vi "SystemNode_Create.vi"(0 "reference":refnum<class "SystemNode.lvclass">, 5 "error in (no error)":errorcluster) -> (14 "reference out":refnum<class "SystemNode.lvclass">, 19 "error out":errorcluster)   [LabVIEW 2016, in "SystemNode.lvclass"]
doc: "Creates and initializes a new SystemNode object.\n\nThis object should be destroyed using a SystemNode destructor VI or a virtual base class destructor VI.\n\n[GOOP 2.1]"
uses:
  <resource>/Framework/Providers/Open_GDS/UML/SystemNode_class/SystemNode.lvclass
  C:/Program Files (x86)/National Instruments/LabVIEW 2016/resource/Framework/Providers/Open_GDS/UML/RectangularNode_class/RectangularNode.lvclass
  <resource>/Framework/Providers/Open_GDS/UML/RectangularNode_class/RectangularNode.lvclass
  <resource>/Framework/Providers/Open_GDS/UML/MultiLineString_class/MultiLineString.lvclass
panel:
  # "The input reference should only\nbe wired when this method is called\nby a sub class constructor."
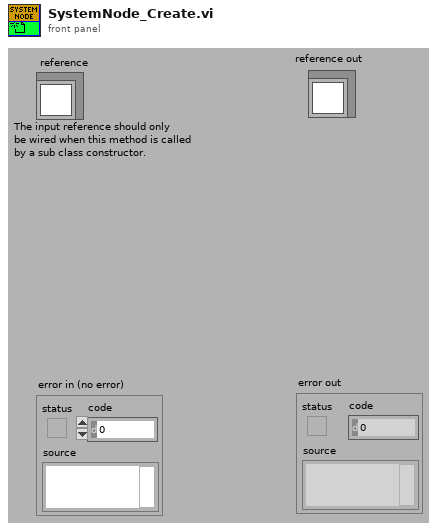
[diagram p1: front panel]
types:
  T1 = typedef "SystemNode.lvclass/ObjectAttributes.ctl" = cluster{"contents":refnum<class "MultiLineString.lvclass">, "DEFAULT_WIDTH":i32, "DEFAULT_HEIGHT":i32, "NAME_GAP":i32, "XGAP":i32, "YGAP":i32}
  T2 = typedef "RectangularNode.lvclass/ObjectAttributes.ctl" = cluster{"bounds":T3}
  T3 = typedef "Rectangle Rectangle2D.ctl" = cluster{"x":dbl, "y":dbl, "width":dbl, "height":dbl}
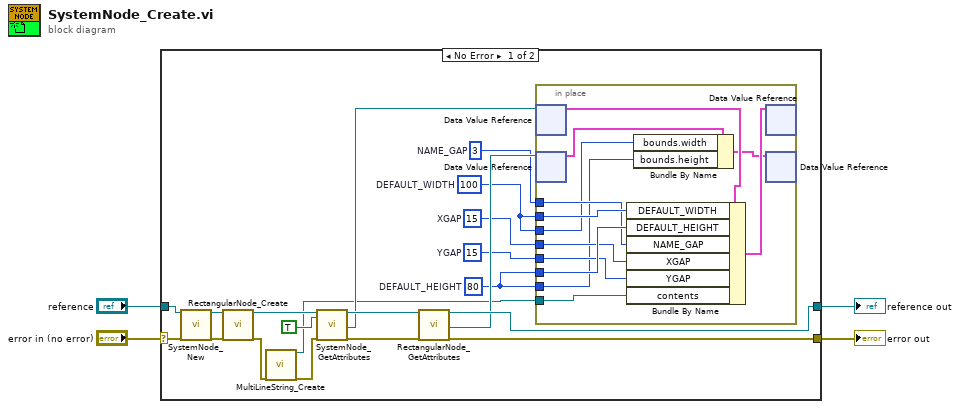
[diagram p0: block diagram]
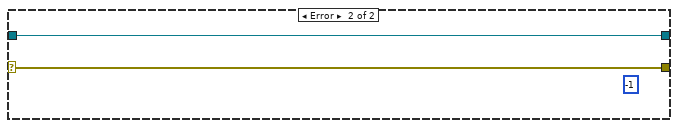
[diagram p2: hidden frame]
diagram:
  n1 = case shown="No Error" "error in (no error)" {
    selector: "error in (no error)" -> [w24 w38]
    tunnel: [w20 w37] -> w4
    tunnel: [w19 w38] -> w3
    tunnel: "reference" -> [w23 w37]
    frame No Error {
      w8 = 15  # YGAP
      w9 = 15  # XGAP
      w10 = 3  # NAME_GAP
      w5 = 80  # DEFAULT_HEIGHT
      w6 = 100  # DEFAULT_WIDTH
      n2 = call <resource>:"SystemNode_New.vi"("reference in"=w23, "error in (no error)"=w24) -> ("reference out"=w21:refnum<class "SystemNode.lvclass">, "error out"=w22:errorcluster)  [unwired: 2 in, 14 out]
      n3 = call <resource>:"RectangularNode_Create.vi"("reference"=w21, "error in (no error)"=w22) -> ("reference out"=w16:refnum<class "SystemNode.lvclass">, "error out"=w18:errorcluster)  [unwired: 1 in, 15 out]
      n4 = call <resource>:"MultiLineString_Create.vi"("error in (no error)"=w18) -> ("reference out"=w7:refnum<class "MultiLineString.lvclass">, "error out"=w17:errorcluster)  [unwired: 2 in, 15 out]
      n5 = call <resource>:"SystemNode_GetAttributes.vi"("reference in"=w16, "OnlyGetDvrReference(False)"=TRUE, "error in (no error)"=w17) -> ("reference out"=w14:refnum<class "SystemNode.lvclass">, "DataRef"=w12:refnum<data-value>, "error out"=w13:errorcluster)  [unwired: 13 in, 1 out]
      n6 = call <resource>:"RectangularNode_GetAttributes.vi"("reference in"=w14, "error in (no error)"=w13) -> ("reference out"=w20:refnum<class "SystemNode.lvclass">, "DataRef"=w11:refnum<data-value>, "error out"=w19:errorcluster)  [unwired: 14 in, 1 out]
      n7 = in-place {
        in-place-border: w6 -> [w35]
        in-place-border: w5 -> [w34]
        in-place-border: w10 -> [w33]
        in-place-border: w9 -> [w32]
        in-place-border: w8 -> [w31]
        in-place-border: w7 -> [w30]
        in-place-border: w6 -> [w27]
        in-place-border: w5 -> [w26]
        n8 = in-place-dvr #1(w12) -> (w36:T1)  [unwired: 1 out]
        n9 = in-place-dvr #2(w11) -> (w28:T2)  [unwired: 1 out]
        n10 = Bundle By Name(cluster=w36, "DEFAULT_WIDTH"=w35, "DEFAULT_HEIGHT"=w34, "NAME_GAP"=w33, "XGAP"=w32, "YGAP"=w31, "contents"=w30) -> (w29:T1)
        n11 = Bundle By Name(cluster=w28, "bounds.width"=w27, "bounds.height"=w26) -> (w25:T2)
        n12 = in-place-dvr #1(w29) -> ()  [unwired: 2 out]
        n13 = in-place-dvr #2(w25) -> ()  [unwired: 2 out]
      }
    }
    frame Error {
      (unwired) -1 ("Nr of open handles")
    }
  }
  "error out" <- w3
  "reference out" <- w4
